vi "Theta Motor Controller.vi"() -> ()   [LabVIEW 2013]
panel:
  in  "stop":bool
  out "Theta Frequency (Hz)":dbl
  in  "Degrees to Move (Deg)":dbl
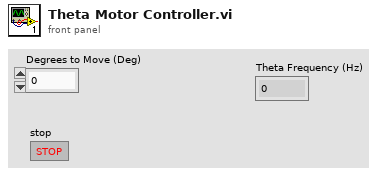
[diagram p1: front panel]
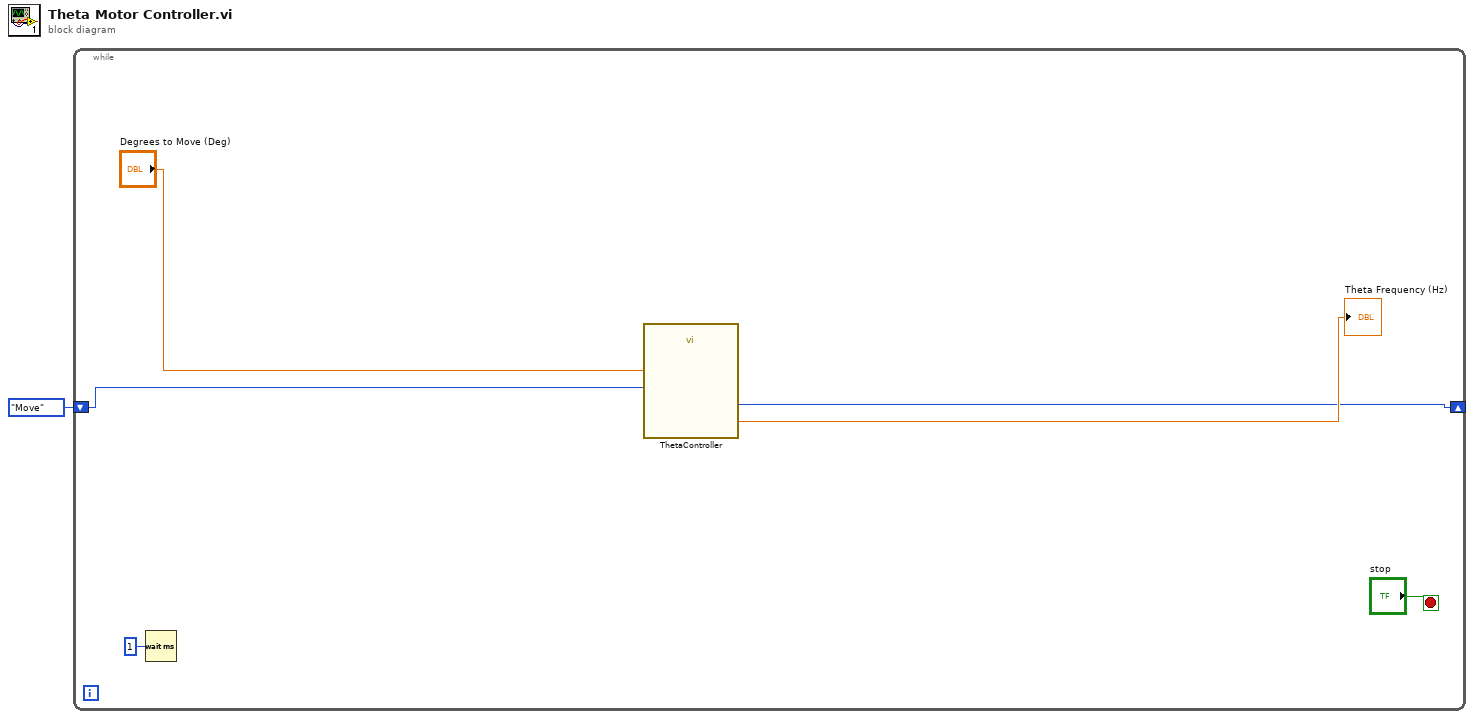
[diagram p0: block diagram]
diagram:
  n1 = while {
    shift-right: [w4] -> _
    shift-left: enum16{"DontMove", "Move"}."Move" ("f") -> [w2]
    stop <- "stop" stop-if-true
    n2 = Wait (ms)(milliseconds to wait=u32 1) -> ()  [unwired: 1 out]
    n3 = call "ThetaController.vi"("Theta Command"=w2, "Degrees to Move (Deg)"="Degrees to Move (Deg)") -> ("Theta Command"=w4:enum16{"DontMove", "Move"}, "Theta Frequency (Hz)"=→"Theta Frequency (Hz)":dbl)  [unwired: 8 in]
  }
